vi "ReadInitCFG.vi"(8 "error in":errorcluster, 9 "UI_EN":bool, 10 "Operation":T2=enum."Read", 11 "CFG":T1={"ProducerEn_PC"=FALSE, "Producer_PC_ms"=0, "ProducerEn_PI"=FALSE, "Producer_PI_ms"=0, "TempLogInterval"=15, "SystemResetTime"=0.0} {"SystemResetTime" format="%<%H:%M:%S>t"}) -> (0 "Error Out":errorcluster, 2 "TempLogInterval[min]":u32, 3 "CFG Out":T1={"ProducerEn_PC"=FALSE, "Producer_PC_ms"=0, "ProducerEn_PI"=FALSE, "Producer_PI_ms"=0, "TempLogInterval"=15, "SystemResetTime"=0.0} {"SystemResetTime" format="%<%H:%M:%S>t"})   [LabVIEW 2020, in "Main.lvlib"]
uses:
  Main.lvlib
  ReadInitCFG/TypeDef/CFG_Cluster.ctl
  ReadInitCFG/TypeDef/Operation.ctl
  <vilib>/Utility/config.llb/NI_LVConfig.lvlib
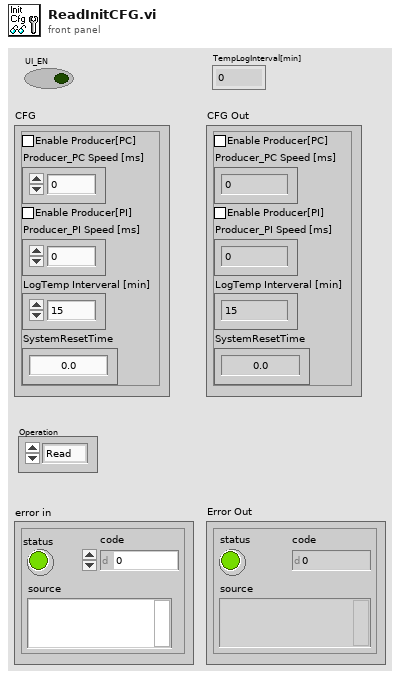
[diagram p1: front panel]
types:
  T1 = typedef "Main.lvlib/CFG_Cluster.ctl" = cluster{"ProducerEn_PC":bool, "Producer_PC_ms":u32, "ProducerEn_PI":bool, "Producer_PI_ms":u32, "TempLogInterval":u32, "SystemResetTime":dbl}
  T2 = typedef "Main.lvlib/Operation.ctl" = enum16{"Write", "Read"}
  T3 = typedef "NI_LVConfig.lvlib/Config Data RefNum.ctl" = refnum<k1>
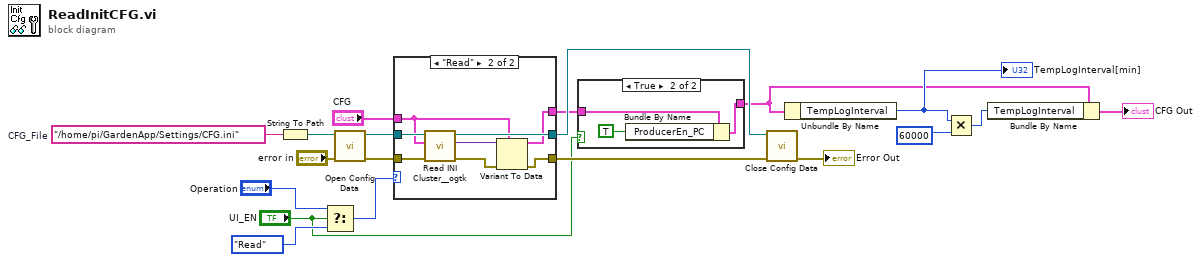
[diagram p0: block diagram]
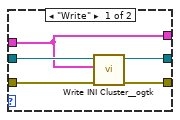
[diagram p3: hidden frame]
diagram:
  w17 = "/home/pi/GardenApp/Settings/CFG.ini"  # CFG_File
  n1 = String To Path(string=w17) -> (path=w18:path)
  n2 = Select(t="Operation", s="UI_EN", f=Operation."Read") -> (s? t:f=w4:T2)
  n3 = call <vilib>:"Open Config Data.vi"("error in (no error)"="error in", "configuration file path"=w18) -> ("error out"=w13:errorcluster, "refnum"=w12:T3)  [unwired: 7 in, 1 out]
  n4 = case shown="\"Read\"" w4 {
    tunnel: w12 -> [w21 w32]
    tunnel: w13 -> [w24 w31]
    tunnel: [w22 w30] -> w14
    tunnel: [w23 w28] -> w15
    tunnel: "CFG" -> [w20 w26]
    tunnel: [w20 w25] -> w3
    frame "Write" {
      n5 = call <userlib>:"Write INI Cluster__ogtk.vi"("error in (no error)"=w24, "INI Fomatted Cluster"=w20, "refnum"=w21) -> ("error out"=w23:errorcluster, "dup refnum"=w22:T3)  [unwired: 7 in]
    }
    frame "Read" {
      n6 = call <userlib>:"Read INI Cluster__ogtk.vi"("error in (no error)"=w31, "INI Fomatted Cluster Type"=w26, "refnum"=w32) -> ("error out"=w29:errorcluster, "INI Fomatted Cluster"=w27:variant, "dup refnum"=w30:T3)  [unwired: 4 in, 2 out]
      n7 = Variant To Data(error in=w29, type=w26, Variant=w27) -> (data=w25:T1, error out=w28:errorcluster)
    }
  }
  n8 = case shown="True" "UI_EN" {
    tunnel: w3 -> [w33 w35]
    tunnel: [w33 w34] -> w2
    frame False {
    }
    frame True {
      n9 = Bundle By Name(cluster=w35, "ProducerEn_PC"=TRUE ("ProducerEn")) -> (w34:T1)
    }
  }
  n10 = call <vilib>:"Close Config Data.vi"("error in (no error)"=w15, "refnum"=w14) -> ("error out"=→"Error Out":errorcluster)  [unwired: 8 in, 1 out]
  n11 = Unbundle By Name(w2) -> ("TempLogInterval"=w8:u32)
  "TempLogInterval[min]" <- w8
  n12 = Multiply(x=w8, y=u32 60000) -> (x*y=w7:u32)
  n13 = Bundle By Name(cluster=w2, "TempLogInterval"=w7) -> (→"CFG Out":T1)
